vi "new FGGA Serial Data Server & Recordingv5.0_10Hz_Scroll_Pump_TCPmillisec.vi"(0 "VISA resource name out":refnum<visa-resource-name>, 11 "error IO":errorcluster) -> ()   [LabVIEW 2014]
uses:
  <vilib>/Platform/TimedLoop/XDataNode/timing_clust.ctl
  <vilib>/Platform/TimedLoop/XDataNode/nitl_modes.ctl
  <vilib>/Platform/TimedLoop/XDataNode/wakeup.ctl
  C:/Program Files (x86)/National Instruments/LabVIEW 2014/examples/Data Communication/Network Streams/Simple Network Streams/support/Network Stream Command.ctl
  <vilib>/Utility/error.llb/whitespace.ctl
  <vilib>/Instr/_visa.llb/VISA Flush IO Buffer Mask.ctl
  <vilib>/Instr/_visa.llb/VISA Configure Serial Port (Instr).vi
  <vilib>/Utility/tcp.llb/UDP Multicast Write-Only Open.vi
  <vilib>/platform/TimedLoop/XDataNode/XDataNode.xnode
  <vilib>/Platform/TimedLoop/XDataNode/XDNodeRunTimeDep.lvlib
panel:
  out "V12":bool
  out "V11":bool
  out "V10":bool
  out "FLOW ALL OFF":bool
  out "LOW FLOW MASTER SWITCH":bool
  out "HIGH FLOW MASTER SWITCH":bool
  out "ASCII_file_out":string
  out "Unix time":u32
  out "FGGA Pump":bool
  out "Flight Number":string
  out "Stop File Write":bool
  out "Default file name":string
  out "MFC":dbl[](array[numeric])
  out "FGGA restart":bool
  out "V4":bool
  out "V3":bool
  out "V2":bool
  out "V1":bool
  out "error out 2":errorcluster
  out "error out":errorcluster
  in  "MFC_1 SLPM set value":dbl
  out "Value Read":string
  out "status":bool
  in  "VISA resource name":refnum<visa-resource-name>="ASRL3::INSTR"
  in  "timeout (10sec) 2":u32=3000
  in  "Clear Display\nErrors":bool
  out "Data Processing":bool
  out "TCP Binary Packet":string
  out "UDP Time Stamp Offset":i32=1
  out "Data String":string
  out "UDP_ACSII_Out":string
  out "Serial error out":errorcluster
  out "SEPTIC TCP Error Out":errorcluster
  out "TCP packet\nSend To SEPTIC":bool
  out "FISH TCP Error Out":errorcluster
  out "TCP packet\nSend To FISH":bool
  out "UDP_Pack_num":u32
  out "UDP_Out Status":bool
  out "UDP_Out_Error Out":errorcluster
  out "Data Array":string[](array[string])
  out "RAW DATA":string
  in  "stop":bool
  out "Number of times \nRead time out":u32
  out "Loop count":i32
  # "Date"
  # "Time"
  # "CH4_wet_ppm"
  # "1"
  # "H2O_ppm"
  # "CO2_wet_ppm"
  # "CH4_dry_ppm"
  # "CO2_dry_ppm"
  # "cell_pressure_torr"
  # "cell_temp_degC"
  # "ambient(bench)_temp_degC"
  # "RDA_us"
  # "RDB_us"
  # "Fitflag"
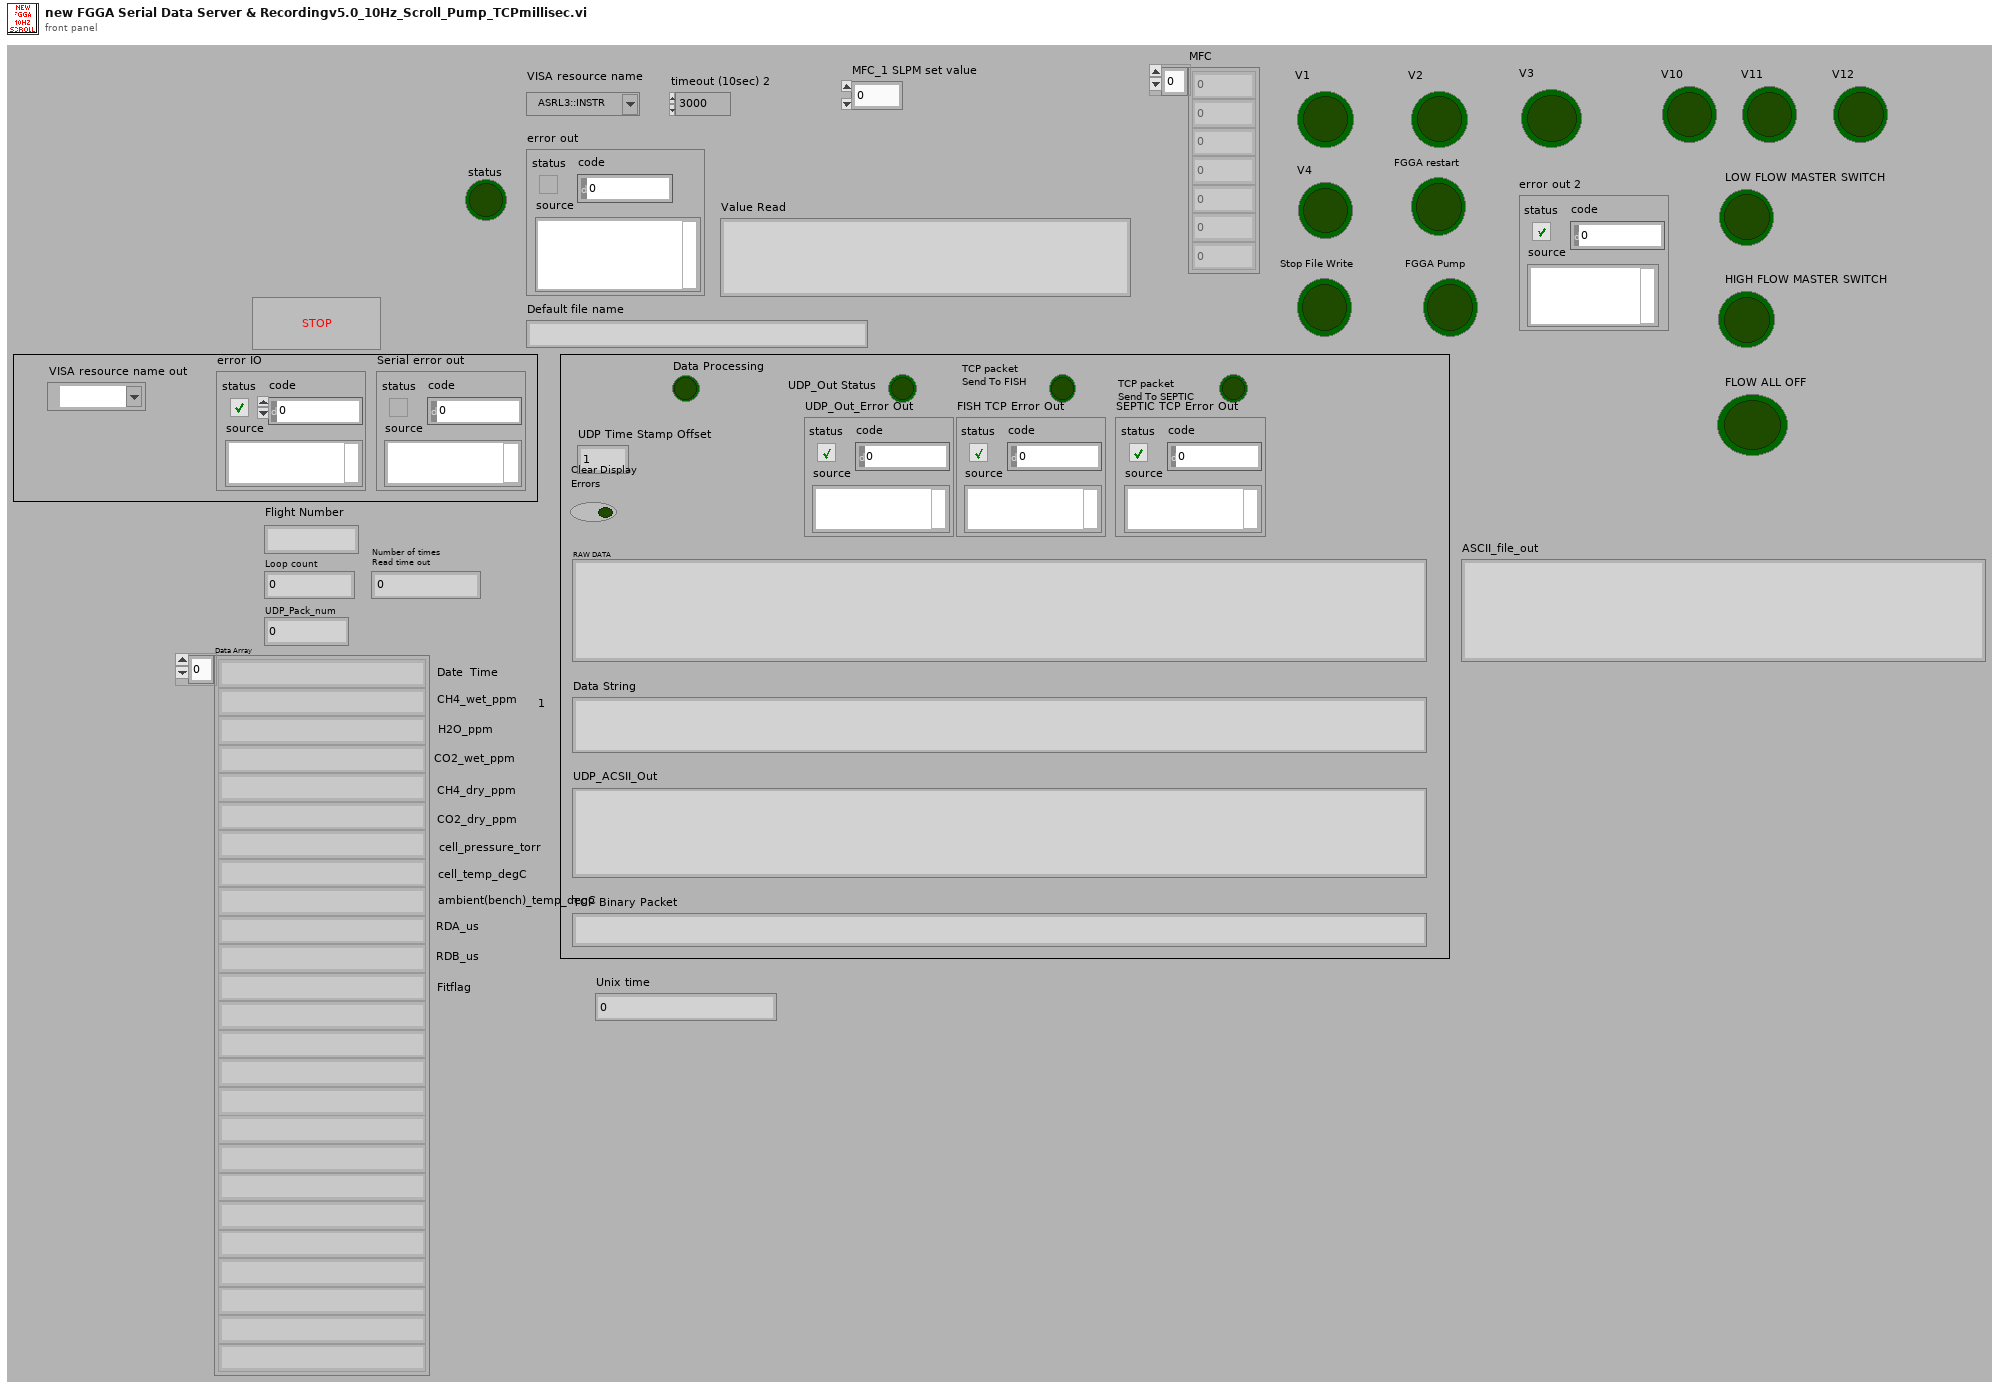
[diagram p1: front panel]
types:
  T1 = typedef "XDNodeRunTimeDep.lvlib/timing_clust.ctl" = cluster{"Expected End [f-1]":u64, "Actual End [f-1]":u64, "Finished Late? [f-1]":bool, "Expected End [i-1]":u64, "Actual End [i-1]":u64, "Finished Late? [i-1]":bool, "Expected Start [i]":u64, "Actual Start [i]":u64, "Expected Start [f]":u64, "Actual Start [f]":u64, "Source Name":string, "Structure Name":string, "Period":i64, "Deadline":i64, "Offset":i64, "Start":i64, "Priority":i32, "Timeout":i32, "Mode":T2, "Wakeup Reason":T3, "Error":errorcluster, "Source Type":string, "Secondary Source Type":string, "Global End Time":u64, "Global Start Time":u64, "Frame Duration":u64, "Iteration Duration":u64, "Assigned CPU":i32, "I/O Scan Engine Mode":u32}
  T2 = typedef "XDNodeRunTimeDep.lvlib/nitl_modes.ctl" = enum32{"No Change", "Process missed periods, maintain original phase", "Discard missed periods, maintain original phase", "Process missed periods, ignore original phase", "Discard missed periods, ignore original phase"}
  T3 = typedef "XDNodeRunTimeDep.lvlib/wakeup.ctl" = enum32{"Normal", "Aborted", "Asynchronous wakeup", "Timing source error", "Timed loop error", "Timeout"}
  T4 = enum16{"open", "replace", "create", "open or create", "replace or create", "replace or create with confirmation"}
  T5 = typedef "Network Stream Command.ctl" = cluster{"Message":string, "Message Data":variant}
  T6 = typedef "whitespace.ctl" = u16
  T7 = typedef "VISA Flush IO Buffer Mask.ctl" = u16
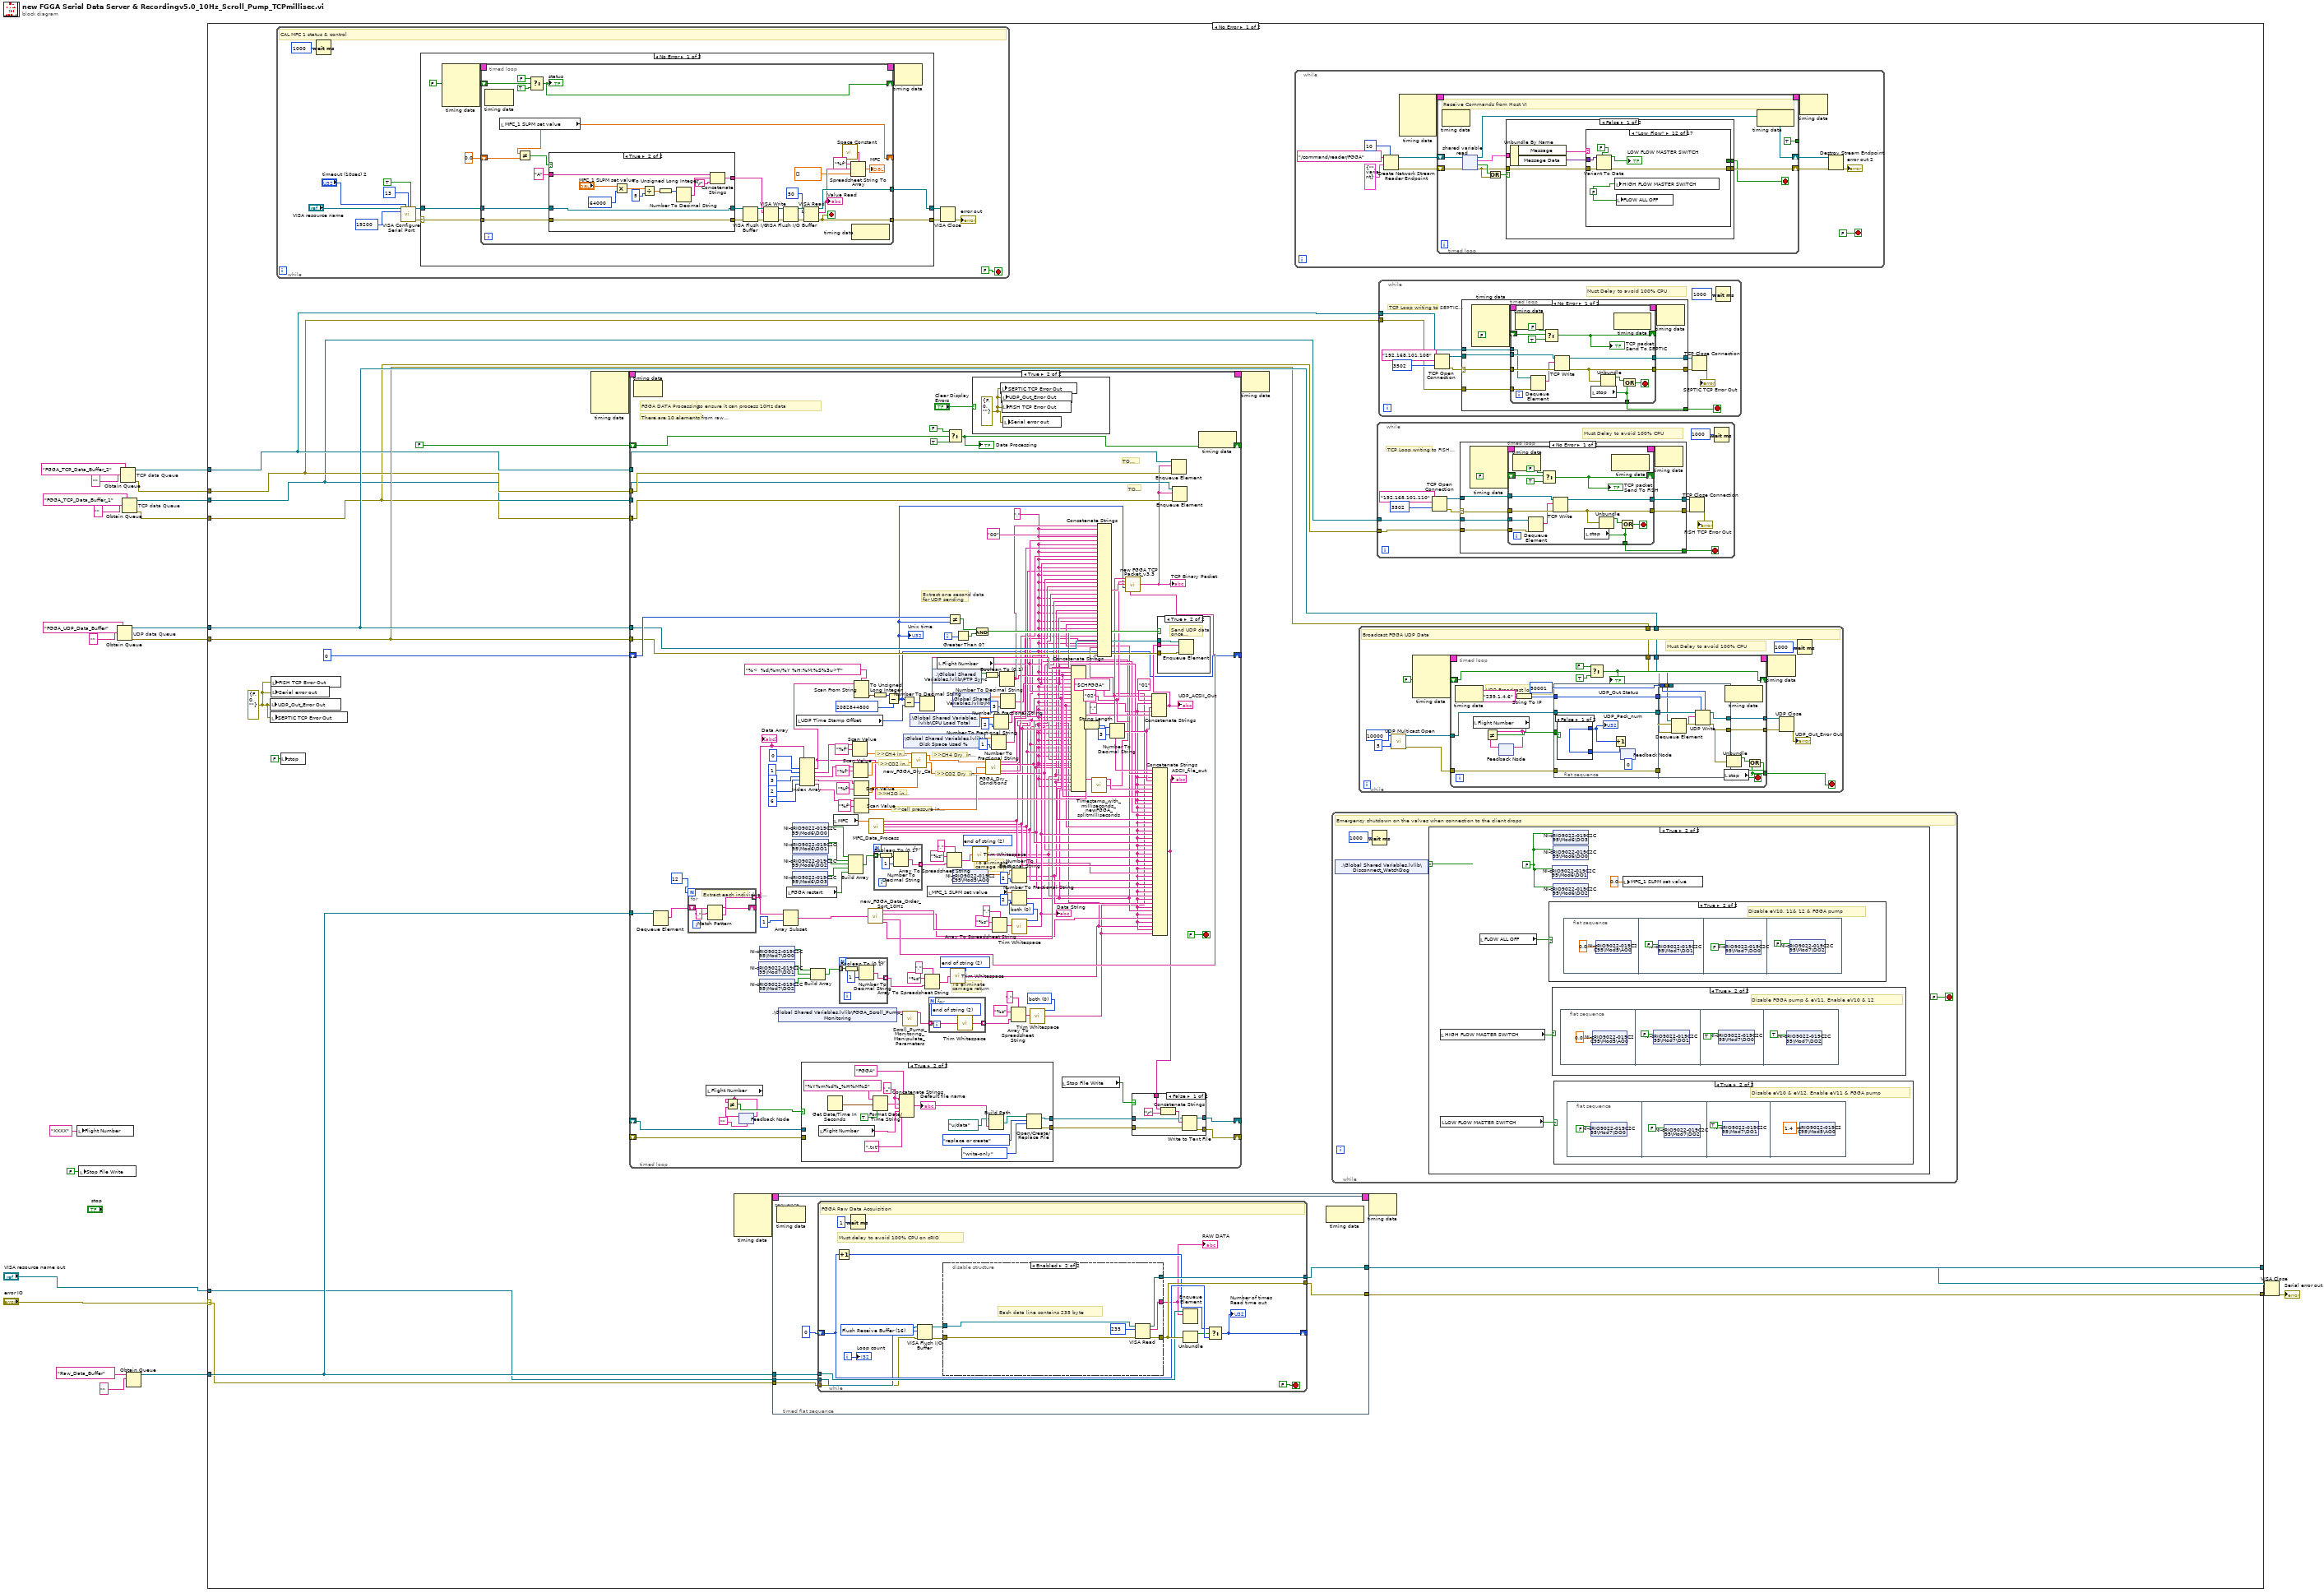
[diagram p0: block diagram]
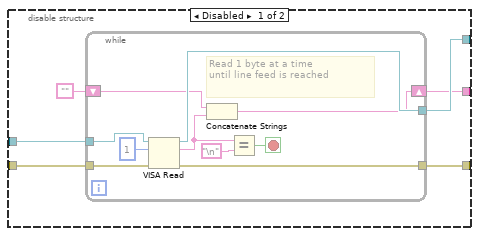
[diagram p2: hidden frame]
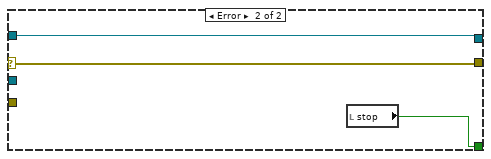
[diagram p3: hidden frame]
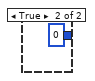
[diagram p4: hidden frame]
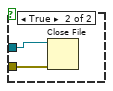
[diagram p6: hidden frame]
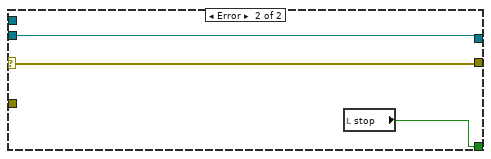
[diagram p9: hidden frame]
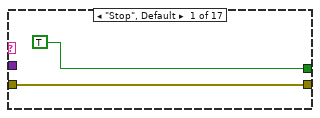
[diagram p14: hidden frame]
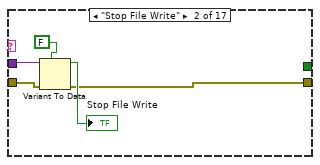
[diagram p15: hidden frame]
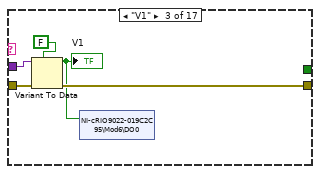
[diagram p16: hidden frame]
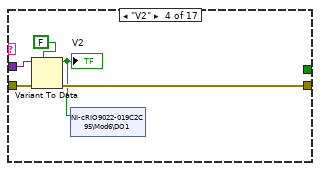
[diagram p17: hidden frame]
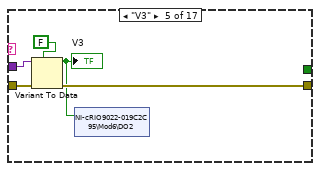
[diagram p18: hidden frame]
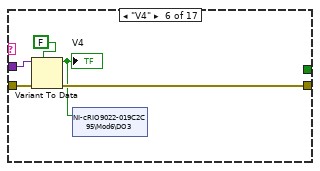
[diagram p19: hidden frame]
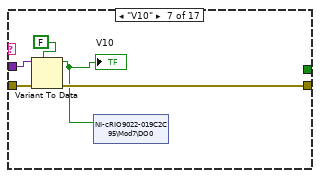
[diagram p20: hidden frame]
diagram:
  n1 = local write "Flight Number"("XXXX" ("Flight Number")) -> ()
  n2 = local write "Stop File Write"(FALSE ("Stop File Write")) -> ()
  n3 = Obtain Queue "UDP data Queue"(name (unnamed)="FGGA_UDP_Data_Buffer", element data type="") -> (queue out=w14:refnum<queue>, error out=w13:errorcluster)  [unwired: 3 in, 1 out]
  n4 = Obtain Queue "TCP data Queue"(name (unnamed)="FGGA_TCP_Data_Buffer_2", element data type="") -> (queue out=w8:refnum<queue>, error out=w7:errorcluster)  [unwired: 3 in, 1 out]
  n5 = Obtain Queue "TCP data Queue"(name (unnamed)="FGGA_TCP_Data_Buffer_1", element data type="") -> (queue out=w6:refnum<queue>, error out=w5:errorcluster)  [unwired: 3 in, 1 out]
  n6 = Obtain Queue(name (unnamed)="Raw_Data_Buffer", element data type="") -> (queue out=w20:refnum<queue>)  [unwired: 3 in, 2 out]
  n7 = case shown="No Error" "error IO" {
    selector: "error IO" -> [w28 w644]
    tunnel: "VISA resource name out" -> [w29 w645]
    tunnel: [w40 w645] -> w17
    tunnel: [w41 w644] -> w18
    tunnel: w20 -> [w39 _]
    tunnel: w14 -> [w37 _]
    tunnel: w13 -> [w36 _]
    tunnel: w8 -> [w35 _]
    tunnel: w7 -> [w34 _]
    tunnel: w6 -> [w33 _]
    tunnel: w5 -> [w32 _]
    frame No Error {
      w25 = errorcluster {"status"=FALSE, "code"=0, "source"=""} ("UDP Error Out")
      n8 = local write "UDP_Out_Error Out"(w25) -> ()
      n9 = local write "SEPTIC TCP Error Out"(w25) -> ()
      n10 = local write "FISH TCP Error Out"(w25) -> ()
      n11 = local write "Serial error out"(w25) -> ()
      n12 = while {
        stop <- FALSE stop-if-true
        # "CAL MFC 1 status & control"
        n13 = Wait (ms)(milliseconds to wait=u32 1000) -> ()  [unwired: 1 out]
        n14 = call-poly "VISA Configure Serial Port"("VISA resource name"="VISA resource name", "timeout (10sec)"="timeout (10sec) 2", "termination char\n(0xA = '\\n' = LF)"=u8 13 ("termination char\n(0xA = '\\n' = LF)"), "Enable Termination\nChar (T)"=TRUE ("Enable Termination\nChar (T)"), "baud rate (9600)"=u32 19200) -> ("VISA resource name out"=w585:refnum<visa-resource-name>, "error out"=w581:errorcluster)  [unwired: 9 in]
        n15 = case shown="No Error" w581 {
          selector: w581 -> [w592 w642]
          tunnel: w585 -> [w593 w643]
          tunnel: [w591 w643] -> w584
          tunnel: [w590 w642] -> w583
          frame No Error {
            n16 = node-c288() -> (w588:T1)  [unwired: 4 in]
            n17 = timed-loop {
              tunnel: w593 -> [w616]
              tunnel: w592 -> [w614]
              tunnel: [w607] -> w591
              tunnel: [w602] -> w590
              shift-right: [w603] -> _
              shift-left: FALSE -> [w606]
              timing: w588 -> [_]
              timing-out: [_] -> w587
              shift-right: [w594] -> _
              shift-left: 0.0 -> [w596]
              stop <- w602 stop-if-true
              n18 = node-c288() -> ()  [unwired: 1 in, 1 out]
              n19 = local read "MFC_1 SLPM set value"() -> (w594:dbl)
              n20 = Not Equal?(x=w594, y=w596) -> (x != y?=w595:bool)
              n21 = Select(t=FALSE, s=w606, f=TRUE) -> (s? t:f=w603:bool)
              "status" <- w603
              n22 = case shown="True" w595 {
                tunnel: w616 -> [w624 w639]
                tunnel: [w624 w639] -> w615
                tunnel: w614 -> [w623 w638]
                tunnel: [w623 w638] -> w613
                tunnel: "A" -> [w627 w631]
                tunnel: [w625 w628] -> w611
                frame False {
                  n23 = Concatenate Strings(w627, "\r") -> (w625:string)
                }
                frame True {
                  n24 = Multiply(x="MFC_1 SLPM set value", y=u32 64000) -> (x*y=w635:dbl)
                  n25 = Divide(x=w635, y=u32 5) -> (x/y=w633:dbl)
                  n26 = To Unsigned Long Integer(number=w633) -> (unsigned 32bit integer=w632:u32)
                  n27 = Number To Decimal String(number=w632) -> (decimal integer string=w630:string)  [unwired: 1 in]
                  n28 = Concatenate Strings(w631, w630, "\r") -> (w628:string)
                }
              }
              n29 = VISA Flush I/O Buffer(VISA resource name=w615, error in (no error)=w613) -> (VISA resource name out=w618:refnum<visa-resource-name>, error out=w617:errorcluster)  [unwired: 1 in]
              n30 = VISA Write(VISA resource name=w618, write buffer=w611, error in (no error)=w617) -> (VISA resource name out=w610:refnum<visa-resource-name>, error out=w609:errorcluster)  [unwired: 1 out]
              n31 = VISA Flush I/O Buffer(VISA resource name=w610, error in (no error)=w609) -> (VISA resource name out=w620:refnum<visa-resource-name>, error out=w619:errorcluster)  [unwired: 1 in]
              n32 = VISA Read(VISA resource name=w620, byte count=u32 50, error in (no error)=w619) -> (VISA resource name out=w607:refnum<visa-resource-name>, read buffer=w601:string, error out=w602:errorcluster)  [unwired: 1 out]
              "Value Read" <- w601
              n33 = call <vilib>:"Space Constant.vi"() -> ("String"=w600:string)
              n34 = Spreadsheet String To Array(delimiter (Tab)=w600, format string="%f", spreadsheet string=w601, array type (2D Dbl)=dbl[] []) -> (array=→"MFC":dbl[])
              n35 = node-c288() -> ()  [unwired: 1 in, 1 out]
            }
            n36 = node-c288(w587) -> ()  [unwired: 1 out]
          }
          frame Error {
          }
        }
        n37 = VISA Close(VISA resource name=w584, error in (no error)=w583) -> (error out=→"error out":errorcluster)
      }
      n38 = local write "stop"(FALSE ("stop")) -> ()
      n39 = node-c288() -> (w27:T1)  [unwired: 4 in]
      n40 = timed-loop {
        timing: w27 -> [_]
        timing-out: [_] -> w26
        tunnel: w39 -> [w341]
        tunnel: w37 -> [w312]
        tunnel: w36 -> [w311]
        shift-right: [w198] -> _
        shift-left: u32 0 -> [w315]
        tunnel: w35 -> [w310]
        tunnel: w34 -> [w309]
        tunnel: w33 -> [w308]
        tunnel: w32 -> [w307]
        shift-right: [w303] -> _
        shift-left: FALSE -> [w306]
        shift-right: [w294] -> _
        shift-left: _ -> [w286]
        shift-right: [w284] -> _
        shift-left: _ -> [w285]
        i -> [w314]
        stop <- FALSE stop-if-true
        w206 = T6 0 items=["both", "start of string", "end of string"] ("location (both)")
        w211 = T6 2 items=["both", "start of string", "end of string"] ("location (both)")
        w260 = T6 2 items=["both", "start of string", "end of string"] ("location (both)")
        w197 = ","
        w330 = T6 0 items=["both", "start of string", "end of string"] ("location (both)")
        w219 = ","
        w242 = "02"
        w243 = "$CHFGGA"
        # "To eliminate\ncarriage return"
        # "To eliminate\ncarriage return"
        # ">>cell pressure in torr>>"
        # "There are 10 elements from raw packet"
        # "TO SEPTIC"
        # "TO FISH"
        # "Extract one second data\nfor UDP sending"
        # ">>CO2 Dry  in ppm>>"
        # ">>CH4 Dry  in ppb>>"
        # ">>H2O in ppm>>"
        # ">>CO2 in ppm>>"
        # ">>CH4 in ppm>>"
        # "Loop Time is 50msec to ensure it can process 10Hz data"
        # "FGGA DATA Processing"
        n41 = node-c288() -> ()  [unwired: 1 in, 1 out]
        n42 = Dequeue Element(queue=w341) -> (element=w302:string)  [unwired: 2 in, 3 out]
        n43 = for {
          N: 12 -> [_]
          shift-right: [w385] -> _
          shift-left: w302 -> [w383]
          tunnel: [w384] -> w335 mode=indexing
          # "Extract each individual param"
          n44 = Match Pattern(string=w383, regular expression=",") -> (before substring=w384:string, after substring=w385:string)  [unwired: 1 in, 2 out]
        }
        "Data Array" <- w335
        n45 = local read "Flight Number"() -> (w283:string)
        n46 = feedback #1("" ("Flight Number")) -> (w291:string)
        n47 = Not Equal?(x=w283, y=w291) -> (x != y?=w289:bool)
        n48 = feedback-in #1(w283) -> ()
        n49 = shared-variable "NI-cRIO9022-019C2C95\\Mod7\\DO1"() -> (w216:bool)  [unwired: 1 in, 1 out]
        n50 = shared-variable "NI-cRIO9022-019C2C95\\Mod7\\DO0"() -> (w217:bool)  [unwired: 1 in, 1 out]
        n51 = shared-variable "NI-cRIO9022-019C2C95\\Mod7\\DO2"() -> (w215:bool)  [unwired: 1 in, 1 out]
        n52 = shared-variable ".\\Global Shared Variables.lvlib\\FGGA_Scroll_Pump_Monitoring"() -> (w204:string[])  [unwired: 1 in, 1 out]
        n53 = Array Subset(array=w335, index=1) -> (w248:string[])  [unwired: 1 in]
        n54 = local read "FGGA restart"() -> (w268:bool)
        n55 = shared-variable "NI-cRIO9022-019C2C95\\Mod6\\DO2"() -> (w274:bool)  [unwired: 1 in, 1 out]
        n56 = shared-variable "NI-cRIO9022-019C2C95\\Mod6\\DO3"() -> (w273:bool)  [unwired: 1 in, 1 out]
        n57 = shared-variable "NI-cRIO9022-019C2C95\\Mod6\\DO0"() -> (w276:bool)  [unwired: 1 in, 1 out]
        n58 = shared-variable "NI-cRIO9022-019C2C95\\Mod6\\DO1"() -> (w275:bool)  [unwired: 1 in, 1 out]
        n59 = local read "UDP Time Stamp Offset"() -> (w259:i32)
        n60 = Index Array(array=w335, index #1=0 ("index"), index #2=1 ("index"), index #3=3 ("index"), index #4=2 ("index"), index #5=6 ("index")) -> (element #1=w238:string, element #2=w254:string, element #3=w253:string, element #4=w252:string, element #5=w251:string)
        n61 = case shown="True" w289 {
          tunnel: [w354 w356] -> w288
          tunnel: [w353 w355] -> w287
          tunnel: w286 -> [w354 _]
          tunnel: w285 -> [w353 _]
          frame False {
          }
          frame True {
            w362 = "_" ("string")
            n62 = local read "Flight Number"() -> (w369:string)
            n63 = Get Date/Time In Seconds() -> (seconds since 1Jan1904=w357:timestamp)
            n64 = Format Date/Time String(time format string (%c)="%Y%m%d%_%H%M%S", seconds (now)=w357, UTC format=TRUE) -> (date/time string=w359:string)
            n65 = Concatenate Strings("FGGA" ("string"), w362, w359, w362, w369, ".txt" ("string")) -> (w364:string)
            "Default file name" <- w364
            n66 = Build Path(base path=path "u:/data", name or relative path=w364) -> (appended path=w368:path)
            n67 = Open/Create/Replace File(file path (use dialog)=w368, operation (0:open)=T4."replace or create", access (0:read/write)=enum16{"read/write", "read-only", "write-only"}."write-only") -> (refnum out=w356:refnum<file>, error out=w355:errorcluster)  [unwired: 3 in, 1 out]
          }
        }
        n68 = Build Array(w217, w216, w215) -> (w218:bool[])
        n69 = local read "MFC"() -> (w295:dbl[])
        n70 = for {
          tunnel: w218 -> [w347] mode=indexing
          tunnel: [w346] -> w210 mode=indexing
          n71 = Boolean To (0,1)(Boolean=w347) -> (0, 1=w348:i16)
          n72 = Number To Decimal String(number=w348, width (-)=i16 1) -> (decimal integer string=w346:string)
        }
        n73 = Build Array(w276, w275, w274, w273, w268) -> (w272:bool[])
        n74 = Scan Value(string=w254, format string="%f") -> (value=w322:dbl)  [unwired: 1 in, 1 out]
        n75 = Scan Value(string=w253, format string="%f") -> (value=w321:dbl)  [unwired: 1 in, 1 out]
        n76 = Scan From String(format string="%<  %d/%m/%Y %H:%M:%S%3u>T", input string=w238) -> (output 1=w199:timestamp)  [unwired: 3 in, 3 out]
        n77 = Scan Value(string=w252, format string="%f") -> (value=w296:dbl)  [unwired: 1 in, 1 out]
        n78 = Scan Value(string=w251, format string="%f") -> (value=w297:dbl)  [unwired: 1 in, 1 out]
        n79 = call "new_FGGA_Data_Order_Sort_10Hz.vi"("Data In"=w248) -> ("UDP Data Out"=w247:string[], "ASCII Ambient(bench)_temp"=w220:string, "TCP Data Out"=w246:string[], "TCP Ambient(bench)_temp"=w245:string)  [unwired: 11 in]
        n80 = call "MFC_Data_Process.vi"("MFC"=w295) -> ("MFC Absolute Pressure"=w228:string, "MFC Temperature"=w227:string, "MFC Volumetric Flow"=w226:string, "MFC Mass Flow"=w225:string, "MFC Set Point"=w224:string)  [unwired: 10 in]
        n81 = To Unsigned Long Integer(number=w199) -> (unsigned 32bit integer=w200:u32)
        n82 = for {
          tunnel: w272 -> [w351] mode=indexing
          tunnel: [w350] -> w269 mode=indexing
          n83 = Boolean To (0,1)(Boolean=w351) -> (0, 1=w352:i16)
          n84 = Number To Decimal String(number=w352, width (-)=i16 1) -> (decimal integer string=w350:string)
        }
        n85 = Subtract(x=w200, y=u32 2082844800) -> (x-y=w198:u32)
        "Unix time" <- w198
        n86 = Subtract(x=w198, y=w259) -> (x-y=w318:u32)
        n87 = call "Scroll_Pump_Monitoring_Manipulate_Parameters.vi"("FGGA_Scroll_Pump\nMonitoring_Input"=w204) -> ("output array"=w203:string[])  [unwired: 14 in]
        n88 = shared-variable ".\\Global Shared Variables.lvlib\\Disk Space Used %"() -> (w262:dbl)  [unwired: 1 in, 1 out]
        n89 = shared-variable ".\\Global Shared Variables.lvlib\\CPU Load Total"() -> (w282:dbl)  [unwired: 1 in, 1 out]
        n90 = call "new_FGGA_Dry_Cal.vi"("H2O"=w296, "CO2_Wet"=w321, "CH4_Wet"=w322) -> ("CO2_Dry"=w299:dbl, "CH4_Dry"=w301:dbl)  [unwired: 7 in]
        n91 = Number To Decimal String(number=w318) -> (decimal integer string=w319:string)  [unwired: 1 in]
        n92 = Array To Spreadsheet String(delimiter (Tab)=",", array=w210, 3:"%s" ("format string")) -> (spreadsheet string=w212:string)
        n93 = local read "MFC_1 SLPM set value"() -> (w264:dbl)
        n94 = for {
          tunnel: w203 -> [w344] mode=indexing
          tunnel: [w343] -> w205 mode=indexing
          w342 = T6 2 items=["both", "start of string", "end of string"] ("location (both)")
          n95 = call <vilib>:"Trim Whitespace.vi"("string"=w344, "location (both)"=w342) -> ("trimmed string"=w343:string)
        }
        n96 = shared-variable ".\\Global Shared Variables.lvlib\\PTP Sync"() -> (w277:bool)  [unwired: 1 in, 1 out]
        n97 = local read "Flight Number"() -> (w234:string)
        n98 = Array To Spreadsheet String(delimiter (Tab)=",", array=w269, 3:"%s" ("format string")) -> (spreadsheet string=w261:string)
        n99 = Select(t=FALSE, s=w306, f=TRUE) -> (s? t:f=w303:bool)
        "Data Processing" <- w303
        n100 = Not Equal?(x=w315, y=w198) -> (x != y?=w316:bool)
        n101 = call <vilib>:"Trim Whitespace.vi"("string"=w212, "location (both)"=w211) -> ("trimmed string"=w202:string)
        n102 = shared-variable ".\\Global Shared Variables.lvlib\\MFM"() -> (w280:dbl)  [unwired: 1 in, 1 out]
        n103 = shared-variable "NI-cRIO9022-019C2C95\\Mod5\\AO0"() -> (w266:dbl)  [unwired: 1 in, 1 out]
        n104 = Greater Than 0?(x=w314) -> (x > 0?=w317:bool)
        n105 = case shown="True" "Clear Display\nErrors" {
          frame False {
          }
          frame True {
            w379 = errorcluster {"status"=FALSE, "code"=0, "source"=""} ("UDP Error Out")
            n106 = local write "SEPTIC TCP Error Out"(w379) -> ()
            n107 = local write "UDP_Out_Error Out"(w379) -> ()
            n108 = local write "FISH TCP Error Out"(w379) -> ()
            n109 = local write "Serial error out"(w379) -> ()
          }
        }
        n110 = call <vilib>:"Trim Whitespace.vi"("string"=w261, "location (both)"=w260) -> ("trimmed string"=w223:string)
        n111 = Compound Arithmetic op=AND(w316, w317) -> (w313:bool)
        n112 = Boolean To (0,1)(Boolean=w277) -> (0, 1=w278:i16)
        n113 = call "FGGA_Dry_Conditions.vi"("CH4_Dry"=w301, "Pressure"=w297, "CO2_Dry"=w299) -> ("CH4_Dry_TCP"=w258:string, "CH4_Dry_UDP"=w230:string, "CO2_Dry_TCP"=w257:string, "CO2_Dry_UDP"=w229:string)  [unwired: 9 in]
        n114 = Number To Fractional String(number=w262, precision (6)=i16 1) -> (F-format string=w232:string)  [unwired: 2 in]
        n115 = Array To Spreadsheet String(delimiter (Tab)=",", array=w247, 3:"%s" ("format string")) -> (spreadsheet string=w329:string)
        n116 = Number To Fractional String(number=w282, precision (6)=i16 2) -> (F-format string=w233:string)  [unwired: 2 in]
        n117 = Number To Decimal String(number=w278) -> (decimal integer string=w236:string)  [unwired: 1 in]
        n118 = Number To Fractional String(number=w280, precision (6)=i16 3) -> (F-format string=w235:string)  [unwired: 2 in]
        n119 = Array To Spreadsheet String(delimiter (Tab)=",", array=w205, 3:"%s" ("format string")) -> (spreadsheet string=w207:string)
        n120 = Number To Fractional String(number=w266, precision (6)=i16 2) -> (F-format string=w222:string)  [unwired: 2 in]
        n121 = Number To Fractional String(number=w264, precision (6)=i16 2) -> (F-format string=w221:string)  [unwired: 2 in]
        n122 = call <vilib>:"Trim Whitespace.vi"("string"=w329, "location (both)"=w330) -> ("trimmed string"=w231:string)
        "Data String" <- w231
        n123 = call <vilib>:"Trim Whitespace.vi"("string"=w207, "location (both)"=w206) -> ("trimmed string"=w201:string)
        n124 = local read "Stop File Write"() -> (w292:bool)
        n125 = Concatenate Strings(w319, w197, w236, w197, w235, w197, w234, w197, w233, w197, w232, w197, w231, w197, w230, w197, w229, w197, w228, w197, w227, w197, w226, w197, w225, w197, w224, w197, w223, w197, w222, w197, w221) -> (w240:string)
        n126 = String Length(string=w240) -> (length=w338:i32)
        n127 = call "Timestamp_with_milliseconds_newFGGA_splitmilliseconds.vi"("Input Time"=w238) -> ("Output Time"=w237:string, "Output split millisecond"=w196:string)  [unwired: 13 in]
        n128 = Concatenate Strings(w236, w197, "00", w197, w234, w197, w258, w197, w257, w197, w235, w197, w228, w197, w227, w197, w226, w197, w225, w197, w224, w197, w223, w197, w222, w197, w221, w197, w245, w197, w202, w197, w201, w197, w196) -> (w256:string)
        n129 = Number To Decimal String(number=w338, width (-)=i16 3) -> (decimal integer string=w241:string)
        n130 = call "new FGGA TCP Packet_v3.3.vi"("ID"=w243, "Version"=w242, "TCP Packet In"=w256, "utc_time"=w198, "Data Array"=w246) -> ("TCP Binary Packet"=w249:string)  [unwired: 10 in]
        "TCP Binary Packet" <- w249
        n131 = Concatenate Strings(w243, "01", w219, w241, w219, w240) -> (w293:string)
        "UDP_ACSII_Out" <- w293
        n132 = Concatenate Strings(w243, w242, w219, w241, w219, w237, w219, w236, w219, w235, w219, w234, w219, w233, w219, w232, w219, w231, w219, w230, w219, w229, w219, w228, w219, w227, w219, w226, w219, w225, w219, w224, w219, w223, w219, w222, w219, w221, w219, w220, w219, w202, w219, w201) -> (w239:string)
        "ASCII_file_out" <- w239
        n133 = case shown="False" w292 {
          tunnel: w239 -> [w376 _]
          tunnel: [w373 _] -> w294
          tunnel: w288 -> [w372 w378]
          tunnel: w287 -> [w371 w377]
          tunnel: [w370 _] -> w284
          frame False {
            n134 = Concatenate Strings(w376, "\r") -> (w374:string)
            n135 = Write to Text File(file (use dialog)=w372, text=w374, error in=w371) -> (refnum out=w373:refnum<file>, error out=w370:errorcluster)  [unwired: 2 out]
          }
          frame True {
            n136 = Close File(refnum=w378, error in=w377) -> ()  [unwired: 2 out]
          }
        }
        n137 = case shown="True" w313 {
          tunnel: w293 -> [_ w382]
          tunnel: w312 -> [_ w381]
          tunnel: w311 -> [_ w380]
          frame False {
          }
          frame True {
            # "Send UDP data once\na second"
            n138 = Enqueue Element(queue=w381, element=w382, error in (no error)=w380) -> ()  [unwired: 1 in, 3 out]
          }
        }
        n139 = Enqueue Element(queue=w310, element=w249, error in (no error)=w309) -> ()  [unwired: 1 in, 3 out]
        n140 = Enqueue Element(queue=w308, element=w249, error in (no error)=w307) -> ()  [unwired: 1 in, 3 out]
        n141 = node-c288() -> ()  [unwired: 1 in, 1 out]
      }
      n142 = node-c288() -> (w24:T1)  [unwired: 4 in]
      n143 = timed-sequence {
        timing: w24 -> [_]
        timing-out: [_] -> w23
        tunnel: [w46] -> w41
        tunnel: [w45] -> w40
        tunnel: w39 -> [w44]
        tunnel: w29 -> [w43]
        tunnel: w28 -> [w42]
        n144 = timed-flat-sequence {
          tunnel: [w52] -> w46
          tunnel: [w51] -> w45
          tunnel: w44 -> [w50]
          tunnel: w43 -> [w49]
          tunnel: w42 -> [w48]
          n145 = node-c288() -> ()  [unwired: 1 in, 1 out]
          n146 = while {
            tunnel: w49 -> [w59]
            tunnel: w48 -> [w58]
            tunnel: [w70] -> w52
            shift-right: [w66] -> _
            shift-left: u32 0 -> [w67]
            tunnel: [w69] -> w51
            tunnel: w50 -> [w64]
            i -> [w68]
            stop <- FALSE stop-if-true
            w55 = T7 16 items=["Flush Receive Buffer"=16, "Write Transmit Buffer to Device"=32, "Flush Receive Buffer (No I/O)"=64, "Flush Transmit Buffer"=128] ("Mask")
            # "Must delay to avoid 100% CPU on cRIO"
            # "FGGA Raw Data Acquisition"
            n147 = Increment(x=w67) -> (x+1=w65:u32)
            n148 = Wait (ms)(milliseconds to wait=u32 1) -> ()  [unwired: 1 out]
            n149 = VISA Flush I/O Buffer(VISA resource name=w59, mask (16)=w55, error in (no error)=w58) -> (VISA resource name out=w56:refnum<visa-resource-name>, error out=w57:errorcluster)
            n150 = disable-structure shown="Enabled" {
              disable-tunnel: [w76 w90] -> w70
              disable-tunnel: [w75 w89] -> w69
              disable-tunnel: [w74 w88] -> w61
              disable-tunnel: w57 -> [w73 w91]
              disable-tunnel: w56 -> [w72 w92]
              frame Disabled {
                n151 = while {
                  tunnel: [w86] -> w75
                  tunnel: [w85] -> w76
                  tunnel: w72 -> [w84]
                  tunnel: w73 -> [w83]
                  shift-right: [w81] -> w74
                  shift-left: "" -> [w82]
                  stop <- w78 stop-if-true
                  # "Read 1 byte at a time \nuntil line feed is reached"
                  n152 = VISA Read(VISA resource name=w84, byte count=u32 1, error in (no error)=w83) -> (VISA resource name out=w86:refnum<visa-resource-name>, read buffer=w80:string, error out=w85:errorcluster)  [unwired: 1 out]
                  n153 = Concatenate Strings(w82, w80) -> (w81:string)
                  n154 = Equal?(x=w80, y="\n") -> (x = y?=w78:bool)
                }
              }
              frame Enabled {
                # "Each data line contains 235 byte"
                n155 = VISA Read(VISA resource name=w92, byte count=u32 235, error in (no error)=w91) -> (VISA resource name out=w89:refnum<visa-resource-name>, read buffer=w88:string, error out=w90:errorcluster)  [unwired: 1 out]
              }
            }
            "RAW DATA" <- w61
            n156 = Enqueue Element(queue=w64, element=w61) -> ()  [unwired: 2 in, 3 out]
            n157 = Unbundle(w70) -> ("status"=w63:bool)  [unwired: 2 out]
            n158 = Select(t=w65, s=w63, f=w67) -> (s? t:f=w66:u32)
            "Number of times \nRead time out" <- w66
            "Loop count" <- w68
          }
          n159 = node-c288() -> ()  [unwired: 1 in, 1 out]
        }
      }
      n160 = node-c288(w26) -> ()  [unwired: 1 out]
      n161 = while {
        stop <- FALSE stop-if-true
        n162 = Create Network Stream Reader Endpoint(7:10 ("reader buffer size"), 9:T5 {"Message"="", "Message Data"=variant} ("Message Cluster"), 11:"/command/reader/FGGA" ("reader url")) -> (0:w459:errorcluster, 3:w460:refnum<k21>)  [unwired: 4 in]
        n163 = node-c288() -> (w454:T1)  [unwired: 4 in]
        n164 = timed-loop "Host->Target Command Reader" {
          shift-right: [w470] -> w457
          shift-left: w459 -> [w473]
          shift-right: [w471] -> w456
          shift-left: w460 -> [w472]
          tunnel: [TRUE] -> _
          timing: w454 -> [_]
          timing-out: [_] -> w453
          stop <- w464 stop-if-true
          # "Receive Commands from Host VI"
          n165 = node-c288() -> ()  [unwired: 1 in, 1 out]
          n166 = shared-variable-read(w472, w473) -> (w471:refnum<k21>, w466:errorcluster, w468:bool, w469:T5)  [unwired: 1 in]
          n167 = Or(x=w468, y=w466) -> (x .or. y?=w467:bool)
          n168 = case shown="False" w467 {
            selector: w467 -> [_ w570]
            tunnel: w466 -> [w481 w571]
            tunnel: [w480 w571] -> w470
            tunnel: w469 -> [w478 _]
            tunnel: [w479 w570] -> w464
            frame False {
              n169 = Unbundle By Name(w478) -> ("Message"=w477:string, "Message Data"=w476:variant)
              n170 = case shown="\"Low_Flow\"" w477 {
                tunnel: w481 -> [w483 w488 w493 w498 w503 w508 w513 w518 w523 w529 w535 w541 w546 w551 w556 w564 w569]
                tunnel: [w483 w484 w492 w497 w502 w507 w512 w517 w522 w528 w534 w540 w545 w550 w555 w563 w568] -> w480
                tunnel: w476 -> [_ w487 w491 w496 w501 w506 w511 w516 w521 w527 w533 w539 w544 w549 w554 w562 w567]
                tunnel: [TRUE _ _ _ _ _ _ _ _ _ _ _ _ _ _ _ _] -> w479
                frame "Stop", Default {
                }
                frame "Stop File Write" {
                  n171 = Variant To Data(error in=w488, type=FALSE, Variant=w487) -> (data=→"Stop File Write":bool, error out=w484:errorcluster)
                }
                frame "V1" {
                  n172 = Variant To Data(error in=w493, type=FALSE, Variant=w491) -> (data=w489:bool, error out=w492:errorcluster)
                  "V1" <- w489
                  n173 = shared-variable "NI-cRIO9022-019C2C95\\Mod6\\DO0"(w489) -> ()  [unwired: 1 in, 1 out]
                }
                frame "V2" {
                  n174 = Variant To Data(error in=w498, type=FALSE, Variant=w496) -> (data=w494:bool, error out=w497:errorcluster)
                  "V2" <- w494
                  n175 = shared-variable "NI-cRIO9022-019C2C95\\Mod6\\DO1"(w494) -> ()  [unwired: 1 in, 1 out]
                }
                frame "V3" {
                  n176 = Variant To Data(error in=w503, type=FALSE, Variant=w501) -> (data=w499:bool, error out=w502:errorcluster)
                  "V3" <- w499
                  n177 = shared-variable "NI-cRIO9022-019C2C95\\Mod6\\DO2"(w499) -> ()  [unwired: 1 in, 1 out]
                }
                frame "V4" {
                  n178 = Variant To Data(error in=w508, type=FALSE, Variant=w506) -> (data=w504:bool, error out=w507:errorcluster)
                  "V4" <- w504
                  n179 = shared-variable "NI-cRIO9022-019C2C95\\Mod6\\DO3"(w504) -> ()  [unwired: 1 in, 1 out]
                }
                frame "V10" {
                  n180 = Variant To Data(error in=w513, type=FALSE, Variant=w511) -> (data=w509:bool, error out=w512:errorcluster)
                  "V10" <- w509
                  n181 = shared-variable "NI-cRIO9022-019C2C95\\Mod7\\DO0"(w509) -> ()  [unwired: 1 in, 1 out]
                }
                frame "V11" {
                  n182 = Variant To Data(error in=w518, type=FALSE, Variant=w516) -> (data=w514:bool, error out=w517:errorcluster)
                  "V11" <- w514
                  n183 = shared-variable "NI-cRIO9022-019C2C95\\Mod7\\DO1"(w514) -> ()  [unwired: 1 in, 1 out]
                }
                frame "V12" {
                  n184 = Variant To Data(error in=w523, type=FALSE, Variant=w521) -> (data=w519:bool, error out=w522:errorcluster)
                  "V12" <- w519
                  n185 = shared-variable "NI-cRIO9022-019C2C95\\Mod7\\DO2"(w519) -> ()  [unwired: 1 in, 1 out]
                }
                frame "No_Flow" {
                  w524 = FALSE
                  n186 = Variant To Data(error in=w529, type=FALSE, Variant=w527) -> (data=→"FLOW ALL OFF":bool, error out=w528:errorcluster)
                  n187 = local write "LOW FLOW MASTER SWITCH"(w524) -> ()
                  n188 = local write "HIGH FLOW MASTER SWITCH"(w524) -> ()
                }
                frame "High_Flow" {
                  w530 = FALSE
                  n189 = Variant To Data(error in=w535, type=FALSE, Variant=w533) -> (data=→"HIGH FLOW MASTER SWITCH":bool, error out=w534:errorcluster)
                  n190 = local write "LOW FLOW MASTER SWITCH"(w530) -> ()
                  n191 = local write "FLOW ALL OFF"(w530) -> ()
                }
                frame "Low_Flow" {
                  w536 = FALSE
                  n192 = Variant To Data(error in=w541, type=FALSE, Variant=w539) -> (data=→"LOW FLOW MASTER SWITCH":bool, error out=w540:errorcluster)
                  n193 = local write "HIGH FLOW MASTER SWITCH"(w536) -> ()
                  n194 = local write "FLOW ALL OFF"(w536) -> ()
                }
                frame "MFC_1" {
                  n195 = Variant To Data(error in=w546, type=0.0, Variant=w544) -> (data=w542:dbl, error out=w545:errorcluster)
                  n196 = local write "MFC_1 SLPM set value"(w542) -> ()
                }
                frame "FGGA_restart" {
                  n197 = Variant To Data(error in=w551, type=FALSE, Variant=w549) -> (data=→"FGGA restart":bool, error out=w550:errorcluster)
                }
                frame "UDP Time Offset" {
                  n198 = Variant To Data(error in=w556, type=0, Variant=w554) -> (data=→"UDP Time Stamp Offset":i32, error out=w555:errorcluster)
                }
                frame "FGGA_pump" {
                  n199 = Variant To Data(error in=w564, type=FALSE, Variant=w562) -> (data=w559:bool, error out=w563:errorcluster)
                  "FGGA Pump" <- w559
                  n200 = Select(t=1.4 ("f"), s=w559, f=0.0 ("t")) -> (s? t:f=w560:dbl)
                  n201 = shared-variable "NI-cRIO9022-019C2C95\\Mod5\\AO0"(w560) -> ()  [unwired: 1 in, 1 out]
                }
                frame "Flight Number" {
                  n202 = Variant To Data(error in=w569, type="", Variant=w567) -> (data=→"Flight Number":string, error out=w568:errorcluster)
                }
              }
            }
            frame True {
            }
          }
          n203 = node-c288() -> ()  [unwired: 1 in, 1 out]
        }
        n204 = node-c288(w453) -> ()  [unwired: 1 out]
        n205 = Destroy Stream Endpoint(8:w457, 11:w456) -> (0:→"error out 2":errorcluster)
      }
      n206 = while {
        stop <- FALSE stop-if-true
        # "Emergency shutdown on the valves when connection to the client drops"
        n207 = shared-variable ".\\Global Shared Variables.lvlib\\Disconnect_WatchDog"() -> (w433:bool)  [unwired: 1 in, 1 out]
        n208 = Wait (ms)(milliseconds to wait=u32 1000) -> ()  [unwired: 1 out]
        n209 = case shown="True" w433 {
          frame False {
          }
          frame True {
            w440 = FALSE
            n210 = local read "HIGH FLOW MASTER SWITCH"() -> (w437:bool)
            n211 = local read "LOW FLOW MASTER SWITCH"() -> (w438:bool)
            n212 = local read "FLOW ALL OFF"() -> (w436:bool)
            n213 = case shown="True" w436 {
              frame False {
              }
              frame True {
                # "Disable eV10, 11& 12 & FGGA pump"
                n214 = flat-sequence {
                  frame #0 {
                    n215 = shared-variable "NI-cRIO9022-019C2C95\\Mod5\\AO0"(0.0) -> ()  [unwired: 1 in, 1 out]
                  }
                  frame #1 {
                    n216 = shared-variable "NI-cRIO9022-019C2C95\\Mod7\\DO1"(FALSE) -> ()  [unwired: 1 in, 1 out]
                  }
                  frame #2 {
                    n217 = shared-variable "NI-cRIO9022-019C2C95\\Mod7\\DO0"(FALSE) -> ()  [unwired: 1 in, 1 out]
                  }
                  frame #3 {
                    n218 = shared-variable "NI-cRIO9022-019C2C95\\Mod7\\DO2"(FALSE) -> ()  [unwired: 1 in, 1 out]
                  }
                }
              }
            }
            n219 = shared-variable "NI-cRIO9022-019C2C95\\Mod6\\DO1"(w440) -> ()  [unwired: 1 in, 1 out]
            n220 = case shown="True" w437 {
              frame False {
              }
              frame True {
                # "Disable FGGA pump & eV11, Enable eV10 & 12"
                n221 = flat-sequence {
                  frame #0 {
                    n222 = shared-variable "NI-cRIO9022-019C2C95\\Mod5\\AO0"(0.0) -> ()  [unwired: 1 in, 1 out]
                  }
                  frame #1 {
                    n223 = shared-variable "NI-cRIO9022-019C2C95\\Mod7\\DO1"(FALSE) -> ()  [unwired: 1 in, 1 out]
                  }
                  frame #2 {
                    n224 = shared-variable "NI-cRIO9022-019C2C95\\Mod7\\DO0"(TRUE) -> ()  [unwired: 1 in, 1 out]
                  }
                  frame #3 {
                    n225 = shared-variable "NI-cRIO9022-019C2C95\\Mod7\\DO2"(TRUE) -> ()  [unwired: 1 in, 1 out]
                  }
                }
              }
            }
            n226 = shared-variable "NI-cRIO9022-019C2C95\\Mod6\\DO3"(w440) -> ()  [unwired: 1 in, 1 out]
            n227 = shared-variable "NI-cRIO9022-019C2C95\\Mod6\\DO0"(w440) -> ()  [unwired: 1 in, 1 out]
            n228 = shared-variable "NI-cRIO9022-019C2C95\\Mod6\\DO2"(w440) -> ()  [unwired: 1 in, 1 out]
            n229 = case shown="True" w438 {
              frame False {
              }
              frame True {
                # "Disable eV10 & eV12, Enable eV11 & FGGA pump"
                n230 = flat-sequence {
                  frame #0 {
                    n231 = shared-variable "NI-cRIO9022-019C2C95\\Mod7\\DO0"(FALSE) -> ()  [unwired: 1 in, 1 out]
                  }
                  frame #1 {
                    n232 = shared-variable "NI-cRIO9022-019C2C95\\Mod7\\DO2"(FALSE) -> ()  [unwired: 1 in, 1 out]
                  }
                  frame #2 {
                    n233 = shared-variable "NI-cRIO9022-019C2C95\\Mod7\\DO1"(TRUE) -> ()  [unwired: 1 in, 1 out]
                  }
                  frame #3 {
                    n234 = shared-variable "NI-cRIO9022-019C2C95\\Mod5\\AO0"(1.4) -> ()  [unwired: 1 in, 1 out]
                  }
                }
              }
            }
            n235 = local write "MFC_1 SLPM set value"(0.0 ("MFC_1 SLPM set value")) -> ()
          }
        }
      }
      n236 = while {
        tunnel: w37 -> [w139]
        tunnel: w36 -> [w138]
        stop <- w140 stop-if-true
        # "Must Delay to avoid 100% CPU"
        # "Broadcast FGGA UDP Data"
        n237 = call-poly <vilib>:"UDP Multicast Open.vi"("time-to-live (1)"=u16 5, "port"=u16 10000) -> ("error out"=w147:errorcluster, "connection ID"=w148:refnum<k16>)  [unwired: 8 in]
        n238 = node-c288() -> (w150:T1)  [unwired: 4 in]
        n239 = timed-loop {
          tunnel: w148 -> [w171]
          tunnel: w147 -> [w170]
          timing: w150 -> [_]
          timing-out: [_] -> w149
          shift-right: [w159] -> _
          shift-left: FALSE -> [w162]
          tunnel: [w158] -> w142
          tunnel: [w156] -> w141
          tunnel: [w154] -> w140
          tunnel: w139 -> [w152]
          tunnel: w138 -> [w151]
          stop <- w155 stop-if-true
          # "UDP Broadcast loop"
          n240 = node-c288() -> ()  [unwired: 1 in, 1 out]
          n241 = local read "Flight Number"() -> (w153:string)
          n242 = feedback-in #2(w153) -> ()
          n243 = feedback #2() -> (w164:string)  [unwired: 1 in]
          n244 = Not Equal?(x=w153, y=w164) -> (x != y?=w163:bool)
          n245 = String To IP(1:"239.1.4.6" ("name")) -> (0:w168:u32)
          n246 = flat-sequence {
            tunnel: w168 -> [w178]
            tunnel: w170 -> [w179]
            tunnel: w171 -> [w180]
            tunnel: [w180] -> w167
            tunnel: [w179] -> w166
            tunnel: [w178] -> w165
            tunnel: w163 -> [w177]
            tunnel: u16 50001 ("port or service name") -> [w191]
            tunnel: w167 -> [w190]
            tunnel: w166 -> [w189]
            tunnel: w165 -> [w188]
            tunnel: [w187] -> w158
            tunnel: [w186] -> w156
            tunnel: w152 -> [w184]
            tunnel: w151 -> [w183]
            frame #0 {
              n247 = feedback #3(u32 0) -> (w174:u32)
              n248 = case shown="False" w177 {
                tunnel: w174 -> [w181 _]
                tunnel: [w181 u32 0] -> w173
                frame False {
                }
                frame True {
                }
              }
              "UDP_Pack_num" <- w173
              n249 = Increment(x=w173) -> (x+1=w175:u32)
              n250 = feedback-in #3(w175) -> ()
            }
            frame #1 {
              n251 = Dequeue Element(queue=w184, error in (no error)=w183) -> (element=w185:string)  [unwired: 1 in, 3 out]
              n252 = UDP Write(address=w188, port or service name=w191, connection ID=w190, data in=w185, 8:w189) -> (error out=w186:errorcluster, 3:w187:refnum<k16>)  [unwired: 1 in]
            }
          }
          n253 = Select(t=FALSE, s=w162, f=TRUE) -> (s? t:f=w159:bool)
          "UDP_Out Status" <- w159
          n254 = local read "stop"() -> (w154:bool)
          n255 = node-c288() -> ()  [unwired: 1 in, 1 out]
          n256 = Unbundle(w156) -> ("status"=w157:bool)  [unwired: 2 out]
          n257 = Compound Arithmetic op=OR(w157, w154) -> (w155:bool)
        }
        n258 = node-c288(w149) -> ()  [unwired: 1 out]
        n259 = UDP Close(connection ID=w142, 8:w141) -> (error out=→"UDP_Out_Error Out":errorcluster)  [unwired: 1 out]
        n260 = Wait (ms)(milliseconds to wait=u32 1000) -> ()  [unwired: 1 out]
      }
      n261 = node-c288(w23) -> ()  [unwired: 1 out]
      n262 = while {
        tunnel: w33 -> [w97]
        tunnel: w32 -> [w96]
        stop <- w100 stop-if-true
        # "Must Delay to avoid 100% CPU"
        # "TCP Loop writing to FISH Tank"
        n263 = TCP Open Connection(address="192.168.101.110", remote port or service name=u16 3502) -> (connection ID=w103:refnum<k5>, error out=w98:errorcluster)  [unwired: 3 in]
        n264 = case shown="No Error" w98 {
          selector: w98 -> [w108 w135]
          tunnel: w103 -> [w113 w136]
          tunnel: [w112 w136] -> w102
          tunnel: [w111 w135] -> w101
          tunnel: [w110 w134] -> w100
          tunnel: w97 -> [w107 _]
          tunnel: w96 -> [w106 _]
          frame No Error {
            n265 = node-c288() -> (w115:T1)  [unwired: 4 in]
            n266 = timed-loop {
              tunnel: w113 -> [w129]
              tunnel: w108 -> [w128]
              tunnel: [w127] -> w112
              tunnel: [w126] -> w111
              tunnel: [w118] -> w110
              shift-right: [w120] -> _
              shift-left: FALSE -> [w123]
              timing: w115 -> [_]
              timing-out: [_] -> w114
              tunnel: w107 -> [w117]
              tunnel: w106 -> [w116]
              stop <- w124 stop-if-true
              n267 = node-c288() -> ()  [unwired: 1 in, 1 out]
              n268 = Dequeue Element(queue=w117, error in (no error)=w116) -> (element=w119:string)  [unwired: 1 in, 3 out]
              n269 = Select(t=FALSE, s=w123, f=TRUE) -> (s? t:f=w120:bool)
              "TCP packet\nSend To FISH" <- w120
              n270 = TCP Write(connection ID=w129, data in=w119, error in (no error)=w128) -> (connection ID out=w127:refnum<k5>, error out=w126:errorcluster)  [unwired: 1 in, 1 out]
              n271 = local read "stop"() -> (w118:bool)
              n272 = Unbundle(w126) -> ("status"=w125:bool)  [unwired: 2 out]
              n273 = node-c288() -> ()  [unwired: 1 in, 1 out]
              n274 = Compound Arithmetic op=OR(w125, w118) -> (w124:bool)
            }
            n275 = node-c288(w114) -> ()  [unwired: 1 out]
          }
          frame Error {
            n276 = local read "stop"() -> (w134:bool)
          }
        }
        n277 = TCP Close Connection(connection ID=w102, error in (no error)=w101) -> (error out=→"FISH TCP Error Out":errorcluster)  [unwired: 1 in, 1 out]
        n278 = Wait (ms)(milliseconds to wait=u32 1000) -> ()  [unwired: 1 out]
      }
      n279 = while {
        tunnel: w35 -> [w393]
        tunnel: w34 -> [w392]
        stop <- w396 stop-if-true
        # "Must Delay to avoid 100% CPU"
        # "TCP Loop writing to SEPTIC Tank"
        n280 = TCP Open Connection(address="192.168.101.108", remote port or service name=u16 3502) -> (connection ID=w399:refnum<k5>, error out=w394:errorcluster)  [unwired: 3 in]
        n281 = case shown="No Error" w394 {
          selector: w394 -> [w404 w431]
          tunnel: w399 -> [w409 w432]
          tunnel: [w408 w432] -> w398
          tunnel: [w407 w431] -> w397
          tunnel: [w406 w430] -> w396
          tunnel: w393 -> [w403 _]
          tunnel: w392 -> [w402 _]
          frame No Error {
            n282 = node-c288() -> (w411:T1)  [unwired: 4 in]
            n283 = timed-loop {
              tunnel: w409 -> [w425]
              tunnel: w404 -> [w424]
              tunnel: [w423] -> w408
              tunnel: [w422] -> w407
              tunnel: [w414] -> w406
              shift-right: [w416] -> _
              shift-left: FALSE -> [w419]
              timing: w411 -> [_]
              timing-out: [_] -> w410
              tunnel: w403 -> [w413]
              tunnel: w402 -> [w412]
              stop <- w420 stop-if-true
              n284 = node-c288() -> ()  [unwired: 1 in, 1 out]
              n285 = Dequeue Element(queue=w413, error in (no error)=w412) -> (element=w415:string)  [unwired: 1 in, 3 out]
              n286 = Select(t=FALSE, s=w419, f=TRUE) -> (s? t:f=w416:bool)
              "TCP packet\nSend To SEPTIC" <- w416
              n287 = TCP Write(connection ID=w425, data in=w415, error in (no error)=w424) -> (connection ID out=w423:refnum<k5>, error out=w422:errorcluster)  [unwired: 1 in, 1 out]
              n288 = local read "stop"() -> (w414:bool)
              n289 = Unbundle(w422) -> ("status"=w421:bool)  [unwired: 2 out]
              n290 = node-c288() -> ()  [unwired: 1 in, 1 out]
              n291 = Compound Arithmetic op=OR(w421, w414) -> (w420:bool)
            }
            n292 = node-c288(w410) -> ()  [unwired: 1 out]
          }
          frame Error {
            n293 = local read "stop"() -> (w430:bool)
          }
        }
        n294 = TCP Close Connection(connection ID=w398, error in (no error)=w397) -> (error out=→"SEPTIC TCP Error Out":errorcluster)  [unwired: 1 in, 1 out]
        n295 = Wait (ms)(milliseconds to wait=u32 1000) -> ()  [unwired: 1 out]
      }
    }
    frame Error {
    }
  }
  n296 = VISA Close(VISA resource name=w17, error in (no error)=w18) -> (error out=→"Serial error out":errorcluster)
